vi "Begin.vi"(11 "image size":T1=enum."320x240") -> (0 "error out":errorcluster)   [LabVIEW 2013]
doc: "Called before other user functions, this VI is expected to open initial I/O refnums, load in file data, and do all program initialization. Notice that the <B>error out</B> terminal is simply used for data flow. Wiring it to other structures or subVIs ensures that this VI runs first."
uses:
  <vilib>/Rock Robotics/WPI/Camera/WPI_CameraImageSize.ctl
  <vilib>/Rock Robotics/WPI/DriverStation/WPI_DriverStationRobotMode2.ctl
  <vilib>/Rock Robotics/SystemInterfaces/DIO/FPGA_DIOChannel.ctl
  <vilib>/Rock Robotics/SystemInterfaces/DIO/FPGA_DIORelayChannel.ctl
  <vilib>/Rock Robotics/WPI/Relay/WPI_RelayDirection.ctl
  <vilib>/Rock Robotics/SystemInterfaces/AI/FPGA_AIGyroChannel.ctl
  <vilib>/Rock Robotics/SystemInterfaces/AI/FPGA_AIChannel.ctl
  <vilib>/Rock Robotics/SystemInterfaces/Typedef/FPGA_TypedefDigitalModule.ctl
  <vilib>/Rock Robotics/WPI/Joystick/WPI_JoystickDeviceEnum.ctl
  <vilib>/Rock Robotics/WPI/Encoder/WPI_EncoderType.ctl
  <vilib>/Rock Robotics/WPI/CAN/Jaguar/SubVIs/WPI_CANJaguar_ControlMode.ctl
  <vilib>/Rock Robotics/WPI/CAN/Jaguar/SubVIs/WPI_CANJaguar_BrakeCoastMode.ctl
  <vilib>/Rock Robotics/SystemInterfaces/DIO/FPGA_DIOPWMChannel.ctl
  Robot Global Data.vi
  <vilib>/Rock Robotics/WPI/Counter/WPI_CounterDigitalInputToDigitalSource.vi
  <vilib>/Rock Robotics/WPI/Counter/WPI_CounterOpen UpDown Mode.vi
  Globals/Useful Values.vi
  <vilib>/Rock Robotics/WPI/MotorControl/WPI_MotorControlOpenCANJaguar.vi
  <vilib>/Rock Robotics/WPI/MotorControl/WPI_MotorControlOpen Jaguar.vi
  <vilib>/Rock Robotics/WPI/Solenoid/WPI_SolenoidOpenSingle.vi
  <vilib>/Rock Robotics/WPI/Solenoid/WPI_SolenoidChannel.ctl
panel:
  in  "Competition?":bool=TRUE
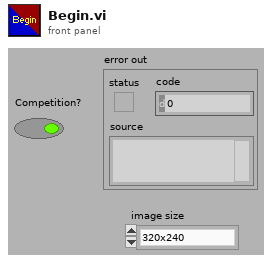
[diagram p1: front panel]
types:
  T1 = typedef "WPI_CameraImageSize.ctl" = enum16{"640x480", "320x240", "160x120"}
  T2 = typedef "FPGA_DIOChannel.ctl" = enum8{"DIO 1", "DIO 2", "DIO 3", "DIO 4", "DIO 5", "DIO 6", "DIO 7", "DIO 8", "DIO 9", "DIO 10", "DIO 11", "DIO 12", "DIO 13", "DIO 14", "Invalid"}
  T3 = typedef "FPGA_DIORelayChannel.ctl" = enum8{"Relay 1", "Relay 2", "Relay 3", "Relay 4", "Relay 5", "Relay 6", "Relay 7", "Relay 8", "Invalid"}
  T4 = typedef "FPGA_DIOPWMChannel.ctl" = enum8{"PWM 1", "PWM 2", "PWM 3", "PWM 4", "PWM 5", "PWM 6", "PWM 7", "PWM 8", "PWM 9", "PWM 10", "Invalid"}
  T5 = typedef "WPI_CANJaguar_BrakeCoastMode.ctl" = enum8{"Jumper", "Brake", "Coast"}
  T6 = typedef "WPI_CANJaguar_ControlMode.ctl" = enum8{"Percent VBus", "Current", "Speed", "Position", "Voltage"}
  T7 = typedef "WPI_RelayDirection.ctl" = enum16{"Both directions", "Forward only", "Reverse only"}
  T8 = typedef "FPGA_AIChannel.ctl" = enum8{"AI 1", "AI 2", "AI 3", "AI 4", "AI 5", "AI 6", "AI 7", "AI 8", "Invalid"}
  T9 = typedef "WPI_EncoderType.ctl" = enum16{"1x", "2x", "4x"}
  T10 = typedef "WPI_JoystickDeviceEnum.ctl" = enum16{"USB 1", "USB 2", "USB 3", "USB 4", "Kinect 1", "Kinect 2"}
  T11 = typedef "FPGA_TypedefDigitalModule.ctl" = enum16{"Digital Module 1", "Digital Module 2"}
  T12 = typedef "FPGA_AIGyroChannel.ctl" = enum8{"AI 1", "AI 2", "Invalid"}
  T13 = typedef "WPI_DriverStationRobotMode2.ctl" = enum16{"Autonomous Disabled", "Autonomous Enabled", "Teleop Disabled", "Teleop Enabled", "Timeout", "Finish", "Test Disabled", "Test Enabled"}
  T14 = typedef "WPI_SolenoidChannel.ctl" = enum8{"Solenoid 1", "Solenoid 2", "Solenoid 3", "Solenoid 4", "Solenoid 5", "Solenoid 6", "Solenoid 7", "Solenoid 8", "Invalid"}
  T15 = typedef "WPI_SolenoidDevRef.ctl" = cluster{"DevStatus":errorcluster, "Solenoid Module":T16, "Forward Solenoid Channel":T14, "Reverse Solenoid Channel":T14}
  T16 = typedef "FPGA_TypedefSolenoidModule.ctl" = enum16{"Solenoid Module 1", "Solenoid Module 2"}
  T17 = typedef "WPI_RelayDevRef.ctl" = cluster{"DevStatus":errorcluster, "Relay Channel":T3, "Digital Module":T11, "Relay Direction":T7}
  T18 = typedef "WPI_CompressorDevRef.ctl" = cluster{"DevStatus":errorcluster, "DigitalInputDevRef":T19, "RelayDevRef":T17}
  T19 = typedef "WPI_DigitalInputDevRef.ctl" = cluster{"DevStatus":errorcluster, "DIO Channel":T2, "Digital Module":T11}
  T20 = typedef "FPGA_CounterEncoderSourceConvertionLVSourceType.ctl" = cluster{"DevStatus":errorcluster, "AnalogTriggerMode?":bool, "DigitalMode":cluster{"Digital Module":T11, "DIO Channel":T21}, "AnalogTriggerMode":cluster{"AnalogTriggerIndex":T22, "OutputType":T23}}
  T21 = typedef "FPGA_DIODigitalSourceChannel.ctl" = enum8{"DIO 1", "DIO 2", "DIO 3", "DIO 4", "DIO 5", "DIO 6", "DIO 7", "DIO 8", "DIO 9", "DIO 10", "DIO 11", "DIO 12", "DIO 13", "DIO 14", "Disabled"}
  T22 = typedef "FPGA_AnalogTriggerIndex.ctl" = enum8{"Trig 0", "Trig 1", "Trig 2", "Trig 3", "Trig 4", "Trig 5", "Trig 6", "Trig 7", "Invalid"}
  T23 = typedef "FPGA_AnalogTriggerOutType.ctl" = enum16{"InWindow", "TriggerState", "Rising", "Falling"}
  T24 = typedef "WPI_MotorControlDeviceRef.ctl" = cluster{"DeviceStatus":errorcluster, "Type":enum16{"PWM", "CAN"}, "PWM":cluster{"Digital Module":T11, "PWM Channel":T4, "DeadBand":T25}, "CAN":cluster{"Device Number":u8, "Control Mode":T6, "Semaphore":T26, "Max Vout":dbl}, "Invert":bool, "TransformRef":T27, "InvTransformRef":T27}
  T25 = typedef "WPI_PWMDeadband.ctl" = cluster{"Name":string, "maxPositivePwm":i32, "minPositivePwm":i32, "centerPwm":i32, "maxNegativePwm":i32, "minNegativePwm":i32, "angularRange":u16}
  T26 = typedef "Semaphore RefNum" = refnum<k1>
  T27 = typedef "WPI_PWMTransform_ConPane.ctl" = refnum<vi>
  T28 = typedef "WPI_EncoderDevRef.ctl" = cluster{"DevStatus":errorcluster, "EncoderIndex":T29, "CounterIndex":T30, "DistancePerCount":dbl, "Decoding Type":T9}
  T29 = typedef "FPGA_EncoderIdx.ctl" = enum8{"Enc 0", "Enc 1", "Enc 2", "Enc 3", "Invalid"}
  T30 = typedef "FPGA_CounterCtrSystemIndex.ctl" = enum8{"Ctr 0", "Ctr 1", "Ctr 2", "Ctr 3", "Ctr 4", "Ctr 5", "Ctr 6", "Ctr 7", "Invalid"}
  T31 = typedef "WPI_JoystickDevRef.ctl" = cluster{"Device":T10}
  T32 = typedef "WPI_CounterDevRef.ctl" = cluster{"DevStatus":errorcluster, "CntIndex":T30}
  T33 = typedef "WPI_DigitalOutputDevRef.ctl" = cluster{"Digital Module":T11, "DIO Channel":T2, "DevStatus":errorcluster}
  T34 = typedef "WPI_GyroDevRef.ctl" = cluster{"DevStatus":errorcluster, "Analog Module":T35, "Analog Channel":T8, "Offset":dbl, "Gain (VoltsPerDegree/Second)":dbl}
  T35 = typedef "FPGA_TypedefAnalogModule.ctl" = enum16{"Analog Module 1", "Analog Module 2"}
  T36 = typedef "WPI_AnalogChannelDevRef.ctl" = cluster{"DevStatus":errorcluster, "Analog Module":T35, "Analog Channel":T8}
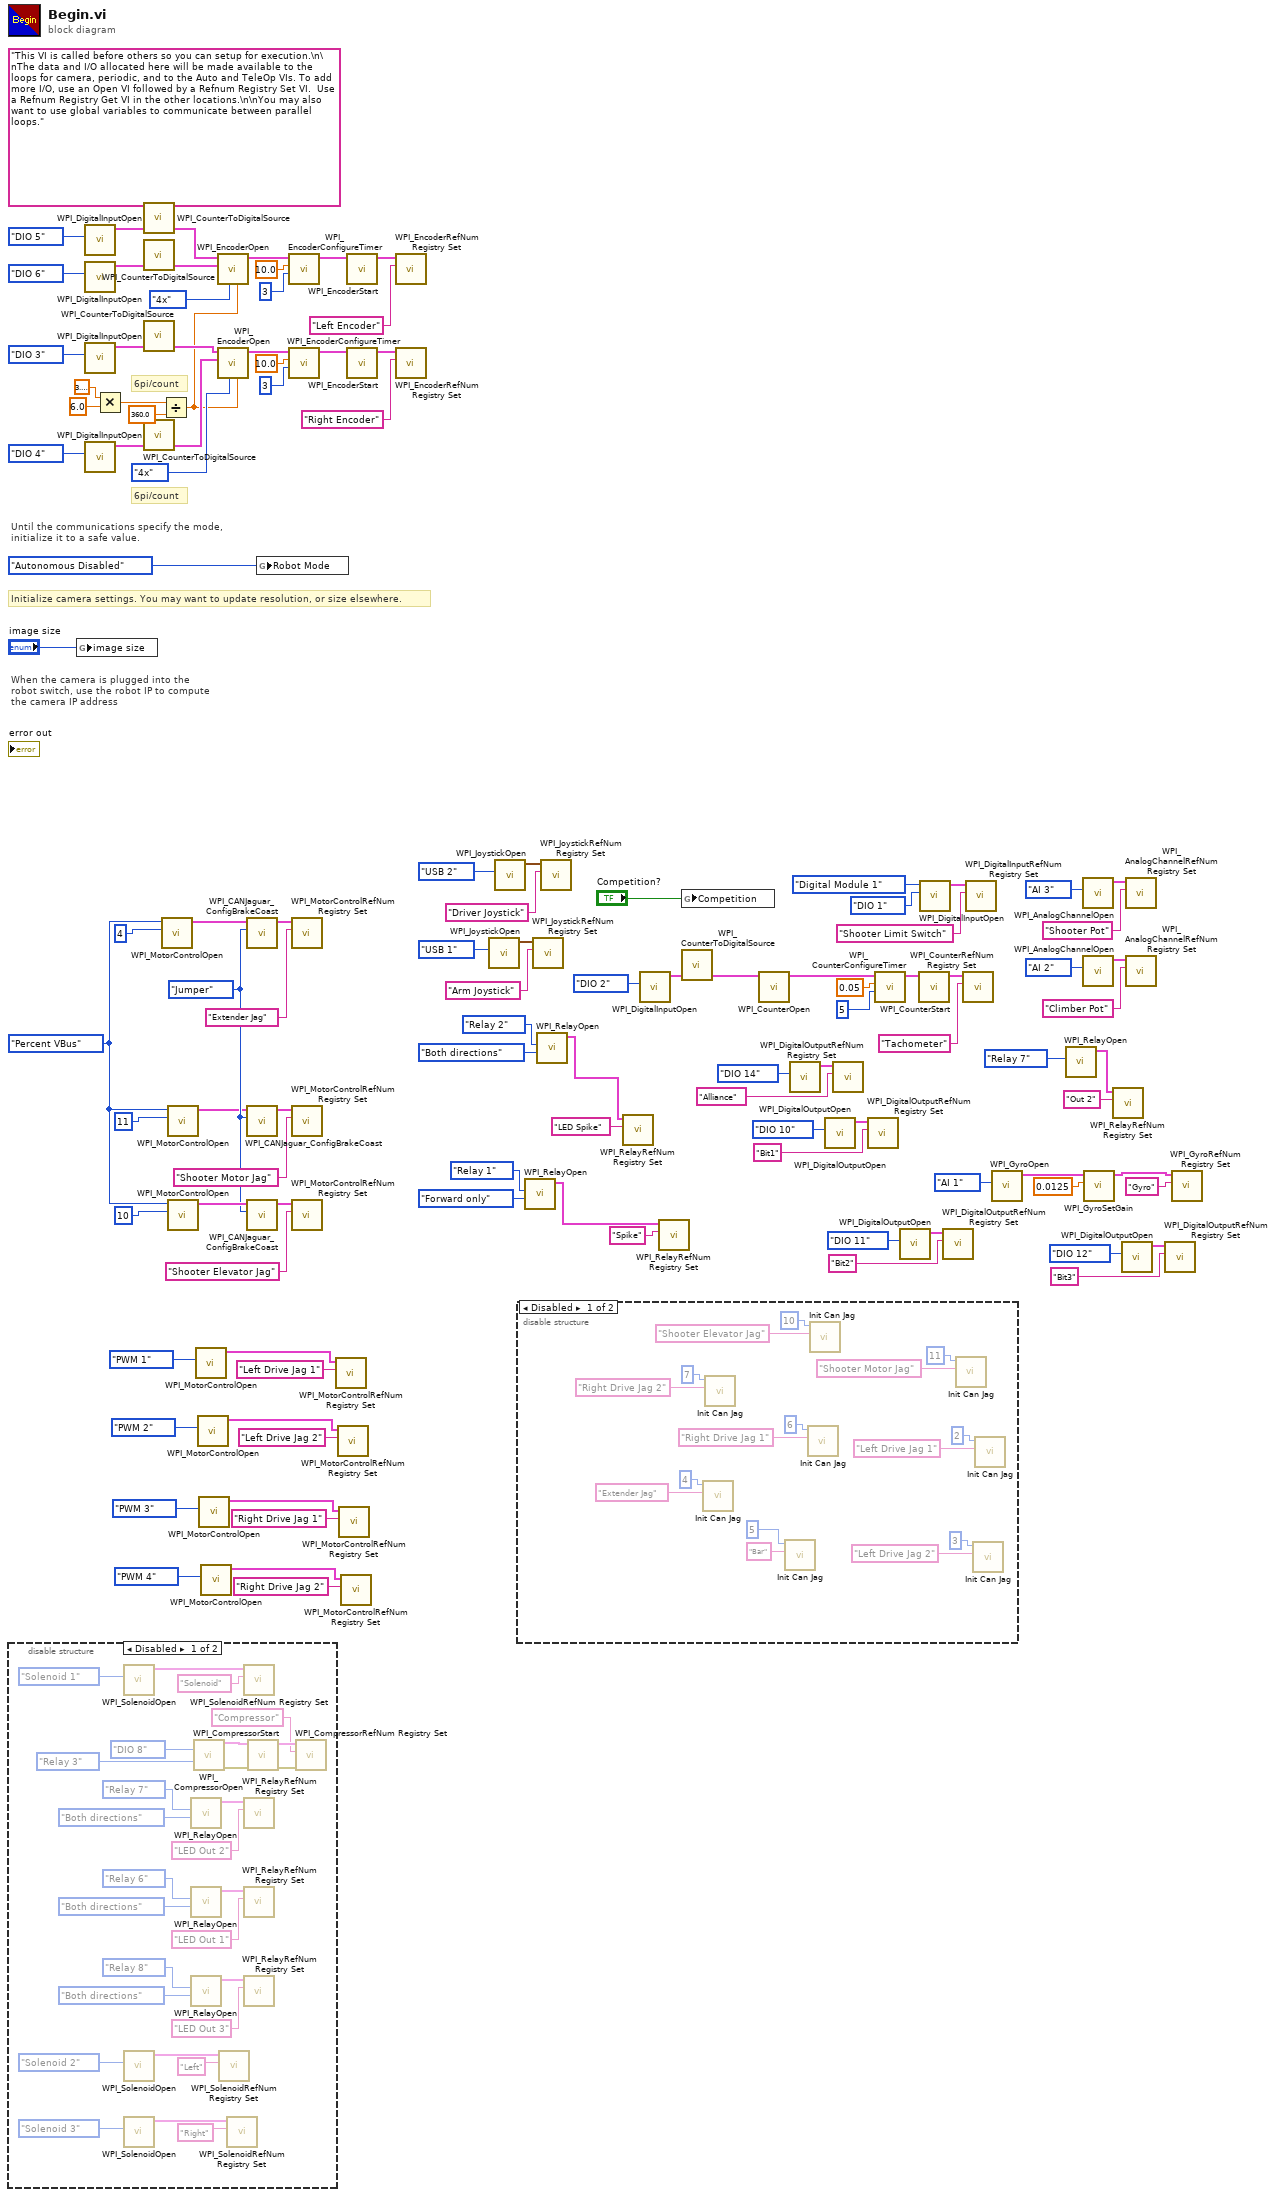
[diagram p0: block diagram]
diagram:
  w29 = WPI_CANJaguar_BrakeCoastMode."Jumper" ("Brake / Coast Mode")
  w30 = WPI_CANJaguar_ControlMode."Percent VBus" ("Control Mode")
  (unwired) "This VI is called before others so you can setup for execution.\n\nThe data and I/O allocated here will be made available to the loops for camera, periodic, and to the Auto and TeleOp VIs. To add more I/O, use an Open VI followed by a Refnum Registry Set VI.  Use a Refnum Registry Get VI in the other locations.\n\nYou may also want to use global variables to communicate between parallel loops."
  # "6pi/count"
  # "6pi/count"
  # "Until the communications specify the mode,\ninitialize it to a safe value."
  # "When the camera is plugged into the\nrobot switch, use the robot IP to compute\nthe camera IP address"
  # "Initialize camera settings. You may want to update resolution, or size elsewhere."
  n1 = disable-structure shown="Disabled" {
    frame Disabled {
      n2 = call-poly <vilib>:"WPI_SolenoidOpen.vi"("Solenoid Channel"=WPI_SolenoidChannel."Solenoid 1") -> ("SolenoidDevRef"=w128:T15)  [unwired: 9 in, 1 out]
      n3 = call-poly <vilib>:"WPI_SolenoidOpen.vi"("Solenoid Channel"=WPI_SolenoidChannel."Solenoid 2") -> ("SolenoidDevRef"=w141:T15)  [unwired: 9 in, 1 out]
      n4 = call-poly <vilib>:"WPI_SolenoidOpen.vi"("Solenoid Channel"=WPI_SolenoidChannel."Solenoid 3") -> ("SolenoidDevRef"=w136:T15)  [unwired: 9 in, 1 out]
      n5 = call <vilib>:"WPI_RelayOpen.vi"("Relay Direction"=WPI_RelayDirection."Both directions", "Relay Channel"=FPGA_DIORelayChannel."Relay 7") -> ("RelayDevRef"=w119:T17)  [unwired: 8 in, 1 out]
      n6 = call <vilib>:"WPI_RelayOpen.vi"("Relay Direction"=WPI_RelayDirection."Both directions", "Relay Channel"=FPGA_DIORelayChannel."Relay 6") -> ("RelayDevRef"=w116:T17)  [unwired: 8 in, 1 out]
      n7 = call <vilib>:"WPI_RelayOpen.vi"("Relay Direction"=WPI_RelayDirection."Both directions", "Relay Channel"=FPGA_DIORelayChannel."Relay 8") -> ("RelayDevRef"=w123:T17)  [unwired: 8 in, 1 out]
      n8 = call <vilib>:"WPI_CompressorOpen.vi"("Pressure Switch DIO Channel"=FPGA_DIOChannel."DIO 8", "Relay Channel"=FPGA_DIORelayChannel."Relay 3") -> ("CompressorDevRef"=w133:T18, "error out"=w129:errorcluster)  [unwired: 12 in]
      n9 = call <vilib>:"WPI_SolenoidRefNum Registry Set.vi"("refnum name"="Left", "SolenoidDevRef"=w141) -> ()  [unwired: 8 in, 2 out]
      n10 = call <vilib>:"WPI_SolenoidRefNum Registry Set.vi"("refnum name"="Right", "SolenoidDevRef"=w136) -> ()  [unwired: 8 in, 2 out]
      n11 = call <vilib>:"WPI_SolenoidRefNum Registry Set.vi"("refnum name"="Solenoid", "SolenoidDevRef"=w128) -> ()  [unwired: 8 in, 2 out]
      n12 = call <vilib>:"WPI_RelayRefNum Registry Set.vi"("refnum name"="LED Out 2", "RelayDevRef"=w119) -> ()  [unwired: 8 in, 2 out]
      n13 = call <vilib>:"WPI_RelayRefNum Registry Set.vi"("refnum name"="LED Out 1", "RelayDevRef"=w116) -> ()  [unwired: 8 in, 2 out]
      n14 = call <vilib>:"WPI_RelayRefNum Registry Set.vi"("refnum name"="LED Out 3", "RelayDevRef"=w123) -> ()  [unwired: 8 in, 2 out]
      n15 = call <vilib>:"WPI_CompressorStart.vi"("error in (no error)"=w129, "CompressorDevRef"=w133) -> ("error out"=w130:errorcluster, "CompressorDevRef"=w135:T18)  [unwired: 8 in]
      n16 = call <vilib>:"WPI_CompressorRefNum Registry Set.vi"("error in (no error)"=w130, "refnum name"="Compressor", "CompressorDevRef"=w135) -> ()  [unwired: 7 in, 2 out]
    }
    frame Enabled {
    }
  }
  n17 = global write "Robot Global Data.vi" "image size"("image size") -> ()
  n18 = call <vilib>:"WPI_DigitalInputOpen.vi"("DIO Channel"=FPGA_DIOChannel."DIO 5") -> ("DigitalInputDevRef"=w62:T19)  [unwired: 9 in, 1 out]
  n19 = call <vilib>:"WPI_DigitalInputOpen.vi"("DIO Channel"=FPGA_DIOChannel."DIO 6") -> ("DigitalInputDevRef"=w61:T19)  [unwired: 9 in, 1 out]
  n20 = call <vilib>:"WPI_DigitalInputOpen.vi"("DIO Channel"=FPGA_DIOChannel."DIO 3") -> ("DigitalInputDevRef"=w60:T19)  [unwired: 9 in, 1 out]
  n21 = call <vilib>:"WPI_DigitalInputOpen.vi"("DIO Channel"=FPGA_DIOChannel."DIO 4") -> ("DigitalInputDevRef"=w59:T19)  [unwired: 9 in, 1 out]
  n22 = Multiply(x=3.141592653589793, y=6.0) -> (x*y=w52:dbl)
  n23 = call-poly <vilib>:"WPI_CounterToDigitalSource.vi"("DigitalInputDevRef"=w62) -> ("Digital Source"=w73:T20)  [unwired: 6 in]
  n24 = call-poly <vilib>:"WPI_CounterToDigitalSource.vi"("DigitalInputDevRef"=w61) -> ("Digital Source"=w72:T20)  [unwired: 6 in]
  n25 = call-poly <vilib>:"WPI_CounterToDigitalSource.vi"("DigitalInputDevRef"=w60) -> ("Digital Source"=w70:T20)  [unwired: 6 in]
  n26 = call-poly <vilib>:"WPI_CounterToDigitalSource.vi"("DigitalInputDevRef"=w59) -> ("Digital Source"=w71:T20)  [unwired: 6 in]
  n27 = Divide(x=w52, y=360.0) -> (x/y=w50:dbl)
  n28 = call-poly <vilib>:"WPI_MotorControlOpen.vi"("Device Number"=u8 4, "Control Mode"=w30) -> ("MotorControlDeviceRef"=w33:T24)  [unwired: 8 in, 1 out]
  n29 = call-poly <vilib>:"WPI_MotorControlOpen.vi"("Device Number"=u8 11, "Control Mode"=w30) -> ("MotorControlDeviceRef"=w28:T24)  [unwired: 8 in, 1 out]
  n30 = call-poly <vilib>:"WPI_MotorControlOpen.vi"("Device Number"=u8 10, "Control Mode"=w30) -> ("MotorControlDeviceRef"=w39:T24)  [unwired: 8 in, 1 out]
  n31 = call-poly <vilib>:"WPI_MotorControlOpen.vi"("PWM Channel"=FPGA_DIOPWMChannel."PWM 1") -> ("MotorControlDeviceRef"=w26:T24)  [unwired: 9 in, 1 out]
  n32 = call-poly <vilib>:"WPI_MotorControlOpen.vi"("PWM Channel"=FPGA_DIOPWMChannel."PWM 2") -> ("MotorControlDeviceRef"=w23:T24)  [unwired: 9 in, 1 out]
  n33 = call-poly <vilib>:"WPI_MotorControlOpen.vi"("PWM Channel"=FPGA_DIOPWMChannel."PWM 3") -> ("MotorControlDeviceRef"=w17:T24)  [unwired: 9 in, 1 out]
  n34 = call-poly <vilib>:"WPI_MotorControlOpen.vi"("PWM Channel"=FPGA_DIOPWMChannel."PWM 4") -> ("MotorControlDeviceRef"=w20:T24)  [unwired: 9 in, 1 out]
  n35 = call <vilib>:"WPI_EncoderOpen.vi"("DistancePerCount"=w50, "Decoding Type"=WPI_EncoderType."4x", "BSource"=w72, "ASource"=w73) -> ("EncoderDevRef"=w80:T28)  [unwired: 6 in, 1 out]
  n36 = call <vilib>:"WPI_EncoderOpen.vi"("DistancePerCount"=w50, "Decoding Type"=WPI_EncoderType."4x", "BSource"=w71, "ASource"=w70) -> ("EncoderDevRef"=w63:T28)  [unwired: 6 in, 1 out]
  n37 = call <vilib>:"WPI_CANJaguar_ConfigBrakeCoast.vi"("Brake / Coast Mode"=w29, "CAN Jaguar Ref"=w33) -> ("CAN Jaguar Ref Out"=w32:T24)  [unwired: 8 in, 1 out]
  n38 = call <vilib>:"WPI_CANJaguar_ConfigBrakeCoast.vi"("Brake / Coast Mode"=w29, "CAN Jaguar Ref"=w28) -> ("CAN Jaguar Ref Out"=w38:T24)  [unwired: 8 in, 1 out]
  n39 = call <vilib>:"WPI_CANJaguar_ConfigBrakeCoast.vi"("Brake / Coast Mode"=w29, "CAN Jaguar Ref"=w39) -> ("CAN Jaguar Ref Out"=w37:T24)  [unwired: 8 in, 1 out]
  n40 = global write "Robot Global Data.vi" "Robot Mode"(WPI_DriverStationRobotMode2."Autonomous Disabled" ("Robot Mode")) -> ()
  n41 = call <vilib>:"WPI_EncoderConfigureTimer.vi"("Number Samples to Average"=u8 3, "Minimum Rate"=10.0, "EncoderDevRef"=w80) -> ("EncoderDevRef"=w79:T28)  [unwired: 7 in, 1 out]
  n42 = call <vilib>:"WPI_EncoderConfigureTimer.vi"("Number Samples to Average"=u8 3, "Minimum Rate"=10.0, "EncoderDevRef"=w63) -> ("EncoderDevRef"=w64:T28)  [unwired: 7 in, 1 out]
  n43 = call <vilib>:"WPI_MotorControlRefNum Registry Set.vi"("refnum name"="Extender Jag", "MotorControlDevRef"=w32) -> ()  [unwired: 8 in, 2 out]
  n44 = call <vilib>:"WPI_MotorControlRefNum Registry Set.vi"("refnum name"="Shooter Motor Jag", "MotorControlDevRef"=w38) -> ()  [unwired: 8 in, 2 out]
  n45 = call <vilib>:"WPI_MotorControlRefNum Registry Set.vi"("refnum name"="Shooter Elevator Jag", "MotorControlDevRef"=w37) -> ()  [unwired: 8 in, 2 out]
  n46 = call <vilib>:"WPI_MotorControlRefNum Registry Set.vi"("refnum name"="Left Drive Jag 1", "MotorControlDevRef"=w26) -> ()  [unwired: 8 in, 2 out]
  n47 = call <vilib>:"WPI_MotorControlRefNum Registry Set.vi"("refnum name"="Left Drive Jag 2", "MotorControlDevRef"=w23) -> ()  [unwired: 8 in, 2 out]
  n48 = call <vilib>:"WPI_MotorControlRefNum Registry Set.vi"("refnum name"="Right Drive Jag 1", "MotorControlDevRef"=w17) -> ()  [unwired: 8 in, 2 out]
  n49 = call <vilib>:"WPI_MotorControlRefNum Registry Set.vi"("refnum name"="Right Drive Jag 2", "MotorControlDevRef"=w20) -> ()  [unwired: 8 in, 2 out]
  n50 = call <vilib>:"WPI_EncoderStart.vi"("EncoderDevRef"=w79) -> ("EncoderDevRef"=w78:T28)  [unwired: 9 in, 1 out]
  n51 = call <vilib>:"WPI_EncoderStart.vi"("EncoderDevRef"=w64) -> ("EncoderDevRef"=w65:T28)  [unwired: 9 in, 1 out]
  n52 = call <vilib>:"WPI_EncoderRefNum Registry Set.vi"("refnum name"="Left Encoder", "EncoderDevRef"=w78) -> ()  [unwired: 8 in, 2 out]
  n53 = call <vilib>:"WPI_EncoderRefNum Registry Set.vi"("refnum name"="Right Encoder", "EncoderDevRef"=w65) -> ()  [unwired: 8 in, 2 out]
  n54 = call <vilib>:"WPI_JoystickOpen.vi"("JoystickDevice"=WPI_JoystickDeviceEnum."USB 1") -> ("JoystickDevRef"=w85:T31)  [unwired: 10 in]
  n55 = call <vilib>:"WPI_JoystickOpen.vi"("JoystickDevice"=WPI_JoystickDeviceEnum."USB 2") -> ("JoystickDevRef"=w86:T31)  [unwired: 10 in]
  n56 = disable-structure shown="Disabled" {
    frame Disabled {
      n57 = call "Init Can Jag.vi"("Motor Name"="Extender Jag" ("refnum name"), "Device Number"=u8 4) -> ()  [unwired: 10 in]
      n58 = call "Init Can Jag.vi"("Motor Name"="Right Drive Jag 2" ("refnum name"), "Device Number"=u8 7) -> ()  [unwired: 10 in]
      n59 = call "Init Can Jag.vi"("Motor Name"="Bar" ("refnum name"), "Device Number"=u8 5) -> ()  [unwired: 10 in]
      n60 = call "Init Can Jag.vi"("Motor Name"="Right Drive Jag 1" ("refnum name"), "Device Number"=u8 6) -> ()  [unwired: 10 in]
      n61 = call "Init Can Jag.vi"("Motor Name"="Shooter Elevator Jag" ("refnum name"), "Device Number"=u8 10) -> ()  [unwired: 10 in]
      n62 = call "Init Can Jag.vi"("Motor Name"="Shooter Motor Jag" ("refnum name"), "Device Number"=u8 11) -> ()  [unwired: 10 in]
      n63 = call "Init Can Jag.vi"("Motor Name"="Left Drive Jag 2" ("refnum name"), "Device Number"=u8 3) -> ()  [unwired: 10 in]
      n64 = call "Init Can Jag.vi"("Motor Name"="Left Drive Jag 1" ("refnum name"), "Device Number"=u8 2) -> ()  [unwired: 10 in]
    }
    frame Enabled {
    }
  }
  n65 = call <vilib>:"WPI_RelayOpen.vi"("Relay Direction"=WPI_RelayDirection."Forward only", "Relay Channel"=FPGA_DIORelayChannel."Relay 1") -> ("RelayDevRef"=w42:T17)  [unwired: 8 in, 1 out]
  n66 = call <vilib>:"WPI_JoystickRefNum Registry Set.vi"("refnum name"="Arm Joystick", "JoystickDevRef"=w85) -> ()  [unwired: 8 in, 2 out]
  n67 = call <vilib>:"WPI_RelayOpen.vi"("Relay Direction"=WPI_RelayDirection."Both directions", "Relay Channel"=FPGA_DIORelayChannel."Relay 2") -> ("RelayDevRef"=w43:T17)  [unwired: 8 in, 1 out]
  n68 = call <vilib>:"WPI_JoystickRefNum Registry Set.vi"("refnum name"="Driver Joystick", "JoystickDevRef"=w86) -> ()  [unwired: 8 in, 2 out]
  n69 = call <vilib>:"WPI_RelayRefNum Registry Set.vi"("refnum name"="LED Spike", "RelayDevRef"=w43) -> ()  [unwired: 8 in, 2 out]
  n70 = call <vilib>:"WPI_DigitalInputOpen.vi"("DIO Channel"=FPGA_DIOChannel."DIO 2") -> ("DigitalInputDevRef"=w112:T19)  [unwired: 9 in, 1 out]
  n71 = call <vilib>:"WPI_RelayRefNum Registry Set.vi"("refnum name"="Spike", "RelayDevRef"=w42) -> ()  [unwired: 8 in, 2 out]
  n72 = global write "Useful Values.vi" "Competition"("Competition?") -> ()
  n73 = call-poly <vilib>:"WPI_CounterToDigitalSource.vi"("DigitalInputDevRef"=w112) -> ("Digital Source"=w96:T20)  [unwired: 6 in]
  n74 = call-poly <vilib>:"WPI_CounterOpen.vi"("Up Source"=w96) -> ("CounterDevRef"=w95:T32)  [unwired: 9 in, 1 out]
  n75 = call <vilib>:"WPI_DigitalOutputOpen.vi"("DIO Channel"=FPGA_DIOChannel."DIO 14") -> ("DigitalOutputDevRef"=w1:T33)  [unwired: 9 in, 1 out]
  n76 = call <vilib>:"WPI_DigitalOutputOpen.vi"("DIO Channel"=FPGA_DIOChannel."DIO 10") -> ("DigitalOutputDevRef"=w6:T33)  [unwired: 9 in, 1 out]
  n77 = call <vilib>:"WPI_DigitalOutputRefNum Registry Set.vi"("refnum name"="Alliance", "DigitalOutputDevRef"=w1) -> ()  [unwired: 8 in, 2 out]
  n78 = call <vilib>:"WPI_DigitalOutputRefNum Registry Set.vi"("refnum name"="Bit1", "DigitalOutputDevRef"=w6) -> ()  [unwired: 8 in, 2 out]
  n79 = call <vilib>:"WPI_CounterConfigureTimer.vi"("Number Samples to Average"=u8 5, "MaxPeriod (sec)"=0.05, "CounterDevRef in"=w95) -> ("CounterDevRef out"=w110:T32)  [unwired: 7 in, 1 out]
  n80 = call <vilib>:"WPI_DigitalOutputOpen.vi"("DIO Channel"=FPGA_DIOChannel."DIO 11") -> ("DigitalOutputDevRef"=w7:T33)  [unwired: 9 in, 1 out]
  n81 = call <vilib>:"WPI_CounterStart.vi"("CounterDevRef in"=w110) -> ("CounterDevRef out"=w94:T32)  [unwired: 9 in, 1 out]
  n82 = call <vilib>:"WPI_DigitalInputOpen.vi"("DIO Channel"=FPGA_DIOChannel."DIO 1", "Digital Module (Module 1)"=FPGA_TypedefDigitalModule."Digital Module 1") -> ("DigitalInputDevRef"=w88:T19)  [unwired: 8 in, 1 out]
  n83 = call <vilib>:"WPI_DigitalOutputRefNum Registry Set.vi"("refnum name"="Bit2", "DigitalOutputDevRef"=w7) -> ()  [unwired: 8 in, 2 out]
  n84 = call <vilib>:"WPI_CounterRefNum Registry Set.vi"("refnum name"="Tachometer", "CounterDevRef"=w94) -> ()  [unwired: 8 in, 2 out]
  n85 = call <vilib>:"WPI_DigitalInputRefNum Registry Set.vi"("refnum name"="Shooter Limit Switch", "DigitalInputDevRef"=w88) -> ()  [unwired: 8 in, 2 out]
  n86 = call <vilib>:"WPI_GyroOpen.vi"("Analog Channel"=FPGA_AIGyroChannel."AI 1") -> ("GyroDevRef"=w104:T34)  [unwired: 8 in, 2 out]
  n87 = call <vilib>:"WPI_RelayOpen.vi"("Relay Channel"=FPGA_DIORelayChannel."Relay 7") -> ("RelayDevRef"=w14:T17)  [unwired: 9 in, 1 out]
  n88 = call <vilib>:"WPI_AnalogChannelOpen.vi"("Analog Channel"=FPGA_AIChannel."AI 3") -> ("AIDeviceRef"=w90:T36)  [unwired: 9 in, 1 out]
  n89 = call <vilib>:"WPI_AnalogChannelOpen.vi"("Analog Channel"=FPGA_AIChannel."AI 2") -> ("AIDeviceRef"=w49:T36)  [unwired: 9 in, 1 out]
  n90 = call <vilib>:"WPI_GyroSetGain.vi"("Gain (VoltsPerDegree/Second)"=0.0125, "GyroDevRef"=w104) -> ("GyroDevRef"=w92:T34)  [unwired: 8 in, 1 out]
  n91 = call <vilib>:"WPI_RelayRefNum Registry Set.vi"("refnum name"="Out 2", "RelayDevRef"=w14) -> ()  [unwired: 8 in, 2 out]
  n92 = call <vilib>:"WPI_DigitalOutputOpen.vi"("DIO Channel"=FPGA_DIOChannel."DIO 12") -> ("DigitalOutputDevRef"=w12:T33)  [unwired: 9 in, 1 out]
  n93 = call <vilib>:"WPI_AnalogChannelRefNum Registry Set.vi"("refnum name"="Shooter Pot", "AIDeviceRef"=w90) -> ()  [unwired: 8 in, 2 out]
  n94 = call <vilib>:"WPI_AnalogChannelRefNum Registry Set.vi"("refnum name"="Climber Pot", "AIDeviceRef"=w49) -> ()  [unwired: 8 in, 2 out]
  n95 = call <vilib>:"WPI_DigitalOutputRefNum Registry Set.vi"("refnum name"="Bit3", "DigitalOutputDevRef"=w12) -> ()  [unwired: 8 in, 2 out]
  n96 = call <vilib>:"WPI_GyroRefNum Registry Set.vi"("refnum name"="Gyro", "GyroDevRef"=w92) -> ()  [unwired: 8 in, 2 out]
